vi "FourFlippingCoins.vi"() -> ()   [LabVIEW 2015]
uses:
  <vilib>/Analysis/NI_AALBase.lvlib
panel:
  out "Waveform Graph":i32[](graph)
  in  "Number of Trials":dbl
  out "Number of Heads":dbl
  out "Coin 4":bool
  out "Coin 3":bool
  out "Coin 2":bool
  out "Coin 1":bool
  # "Heads=Lit"
  # "Tails=Unlit"
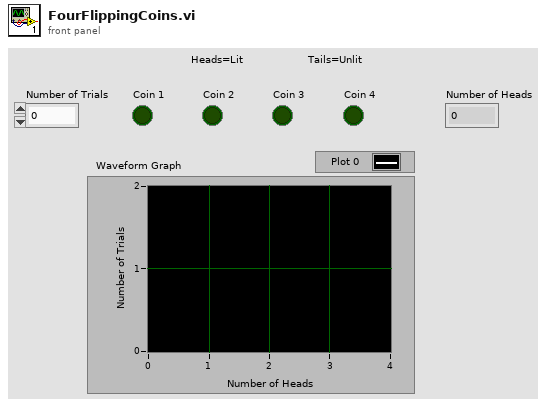
[diagram p1: front panel]
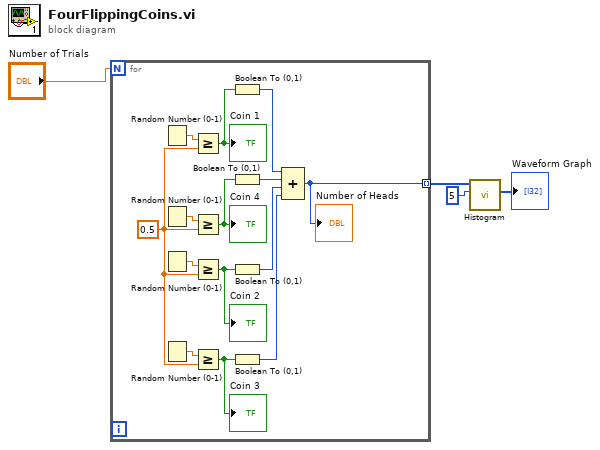
[diagram p0: block diagram]
diagram:
  n1 = for {
    N: "Number of Trials" -> [_]
    tunnel: [w5] -> w2 mode=indexing
    w18 = 0.5
    n2 = Random Number (0-1)() -> (number: 0 to 1=w14:dbl)
    n3 = Random Number (0-1)() -> (number: 0 to 1=w15:dbl)
    n4 = Random Number (0-1)() -> (number: 0 to 1=w16:dbl)
    n5 = Random Number (0-1)() -> (number: 0 to 1=w17:dbl)
    n6 = Greater Or Equal?(x=w14, y=w18) -> (x >= y?=w6:bool)
    "Coin 1" <- w6
    n7 = Greater Or Equal?(x=w15, y=w18) -> (x >= y?=w7:bool)
    "Coin 4" <- w7
    n8 = Greater Or Equal?(x=w16, y=w18) -> (x >= y?=w8:bool)
    "Coin 2" <- w8
    n9 = Greater Or Equal?(x=w17, y=w18) -> (x >= y?=w9:bool)
    "Coin 3" <- w9
    n10 = Boolean To (0,1)(Boolean=w6) -> (0, 1=w10:i16)
    n11 = Boolean To (0,1)(Boolean=w7) -> (0, 1=w12:i16)
    n12 = Boolean To (0,1)(Boolean=w8) -> (0, 1=w13:i16)
    n13 = Boolean To (0,1)(Boolean=w9) -> (0, 1=w11:i16)
    n14 = Compound Arithmetic op=ADD(w10, w12, w13, w11) -> (w5:i16)
    "Number of Heads" <- w5
  }
  n15 = call <vilib>:"Histogram.vi"("intervals"=5, "X"=w2) -> ("Histogram: h(x)"=→"Waveform Graph":i32[])  [unwired: 6 in, 3 out]
